vi "TipShaper_Xsizing_sub.vi"(11 "TipLift":dbl) -> (3 "Text":string)   [LabVIEW 2014]
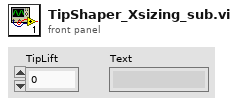
[diagram p1: front panel]
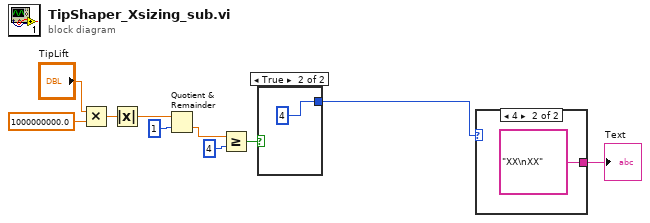
[diagram p0: block diagram]
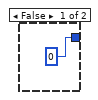
[diagram p2: hidden frame]
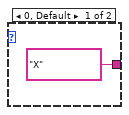
[diagram p3: hidden frame]
diagram:
  n1 = Multiply(x="TipLift", y=1000000000.0) -> (x*y=w3:dbl)
  n2 = Absolute Value(x=w3) -> (abs(x)=w10:dbl)
  n3 = Quotient & Remainder(x=w10, y=1) -> (floor(x/y)=w1:dbl)  [unwired: 1 out]
  n4 = Greater Or Equal?(x=w1, y=4) -> (x >= y?=w7:bool)
  n5 = case shown="True" w7 {
    tunnel: [0 4] -> w2
    frame False {
    }
    frame True {
    }
  }
  n6 = case shown="4" w2 {
    tunnel: ["X" "XX\nXX" ("Text")] -> w6
    frame 0, Default {
    }
    frame 4 {
    }
  }
  "Text" <- w6
